vi "Query IO.vi"(8 "error in":errorcluster, 11 "6512 in":refnum<class "6512.lvclass">) -> (0 "error out":errorcluster, 1 "Port Array":u8[](array[numeric]), 2 "Boolean Array":bool[](array[boolean]), 3 "6512 out":refnum<class "6512.lvclass">)   [LabVIEW 2019, in "6512.lvlib" / "6512.lvclass"]
doc: "This method must be overridden by the child class.\n\nThis should read the status at the output of the device and return a weform capture of the named signal states."
uses:
  Library/6512.lvclass
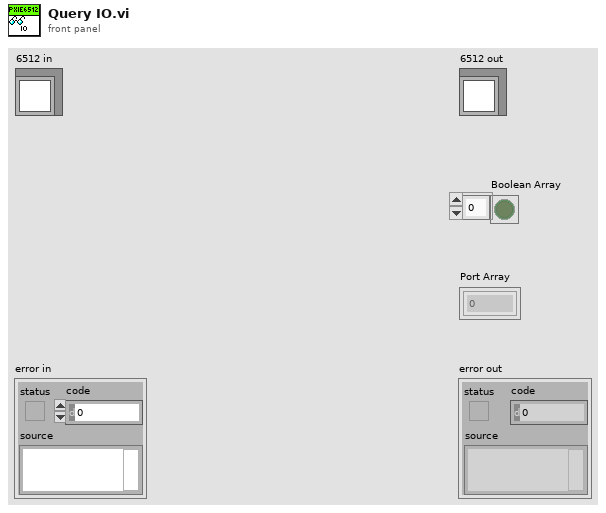
[diagram p1: front panel]
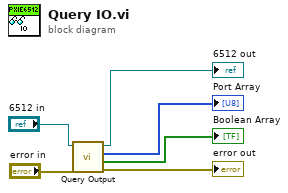
[diagram p0: block diagram]
diagram:
  n1 = call "Query Output.vi"("error in"="error in", "6512 in"="6512 in") -> ("error out"=→"error out":errorcluster, "Boolean array"=→"Boolean Array":bool[], "Port Array"=→"Port Array":u8[], "6512 out"=→"6512 out":refnum<class "6512.lvclass">)  [unwired: 6 in]
